vi "Actor Main.vi"(9 "Root Actor Address":refnum<class "Mail Strategy.lvclass">, 11 "System Actor Obj":refnum<class "System Actor.lvclass">) -> ()   [LabVIEW 2024]
uses:
  System Actor/System Actor.lvclass
  Messenger/Mail Strategy/Mail Strategy.lvclass
  System Actor/System Actor.lvclass/System Actor.ctl
  System Actor/Public Data/Read IDs.vi
  Polymorphic VIs/Converter/1D I64 To String with Interval.vi
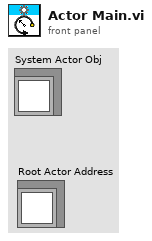
[diagram p1: front panel]
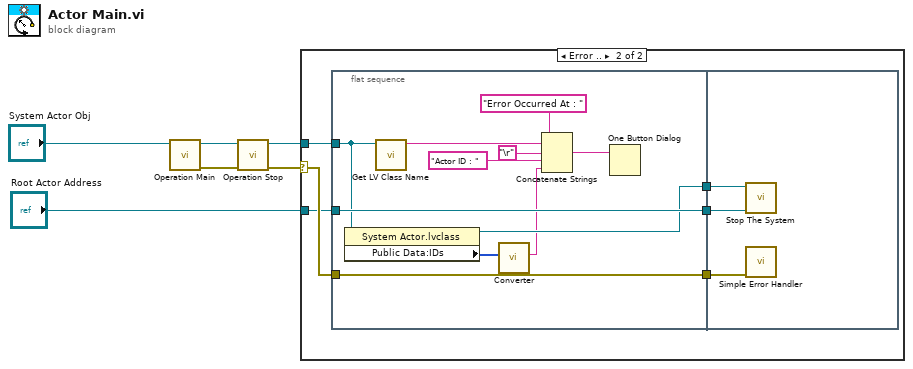
[diagram p0: block diagram]
diagram:
  n1 = call-dynamic "Operation Main.vi"("System Actor in"="System Actor Obj") -> ("error out"=w4:errorcluster, "System Actor out"=w5:refnum<class "System Actor.lvclass">)  [unwired: 9 in]
  n2 = call-dynamic "Operation Stop.vi"("error in (no error)"=w4, "System Actor in"=w5) -> ("error out"=w3:errorcluster, "System Actor out"=w2:refnum<class "System Actor.lvclass">)  [unwired: 8 in]
  n3 = case shown="Error .." w3 {
    selector: w3 -> [_ w10]
    tunnel: w2 -> [_ w12]
    tunnel: "Root Actor Address" -> [_ w7]
    frame No Error {
    }
    frame Error {
      n4 = flat-sequence {
        tunnel: w12 -> [w18]
        tunnel: [w20] -> w11
        tunnel: w10 -> [w20]
        tunnel: [w15] -> w9
        tunnel: [w19] -> w8
        tunnel: w7 -> [w19]
        tunnel: w11 -> [w26]
        tunnel: w9 -> [w25]
        tunnel: w8 -> [w24]
        frame #0 {
          n5 = property class="System Actor.lvclass"(reference=w18) -> (reference out=w15:refnum<class "System Actor.lvclass">, "Public Data:IDs"=w14:i64[])  [unwired: 1 in, 1 out]
          n6 = call <vilib>:"Get LV Class Name.vi"("object"=w18) -> ("class name"=w23:string)  [unwired: 9 in, 1 out]
          n7 = call-poly "Converter.vi"("Array In"=w14) -> ("String out"=w13:string)  [unwired: 10 in]
          n8 = Concatenate Strings("Error Occurred At : " ("string"), w23, "\r", "Actor ID : " ("string"), w13) -> (w21:string)
          n9 = One Button Dialog(message=w21) -> ()  [unwired: 1 in, 1 out]
        }
        frame #1 {
          n10 = call "Stop The System.vi"("Root Actor Address"=w24, "System Actor in"=w25) -> ()  [unwired: 9 in, 1 out]
          n11 = call <vilib>:"Simple Error Handler.vi"("error in (no error)"=w26) -> ()  [unwired: 4 in, 5 out]
        }
      }
    }
  }
